vi "Omron_COMM_Initial.vi"(8 "error in":errorcluster, 11 "COM in":refnum<visa-resource-name>) -> (0 "error out":errorcluster, 3 "COM out":refnum<visa-resource-name>)   [LabVIEW 2017]
uses:
  <vilib>/Instr/_visa.llb/VISA Configure Serial Port (Instr).vi
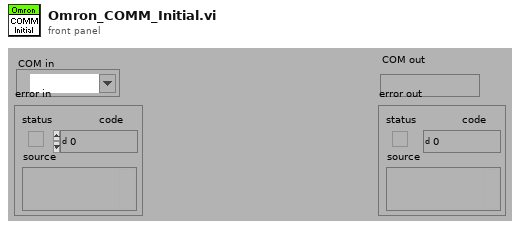
[diagram p1: front panel]
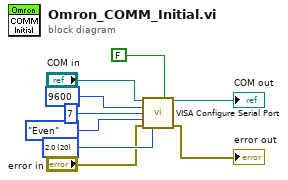
[diagram p0: block diagram]
diagram:
  w5 = u16 20 items=["1.0"=10, "1.5"=15, "2.0"=20] ("stop bits (10: 1 bit)")
  n1 = call-poly "VISA Configure Serial Port"("VISA resource name"="COM in", "Enable Termination\nChar (T)"=FALSE ("Enable Termination\nChar (T)"), "baud rate (9600)"=u32 9600, "data bits (8)"=u16 7, "parity (0:none)"=enum16{"None", "Odd", "Even", "Mark", "Space"}."Even", "error in (no error)"="error in", "stop bits (10: 1 bit)"=w5) -> ("VISA resource name out"=→"COM out":refnum<visa-resource-name>, "error out"=→"error out":errorcluster)  [unwired: 7 in]
